vi "Configure Set Vol.vi"(8 "error in (no error)":errorcluster, 9 "Voltage set (0.00 V)":dbl format="%.2g", 10 "Ch Selector":T1, 11 "VISA resource name":refnum<visa-resource-name>) -> (0 "error out":errorcluster, 3 "VISA resource name out":refnum<visa-resource-name>)   [LabVIEW 2020, in "ScientiFic DC Power Supply.lvlib"]
doc: "Configures Set voltage of the power supply. Specify the set voltage limit for Your Application"
uses:
  <instrlib>/ScientiFic DC Power Supply/ScientiFic DC Power Supply.lvlib
  <instrlib>/ScientiFic DC Power Supply/Public/Ch Selector.ctl
panel:
  out "read buffer":string
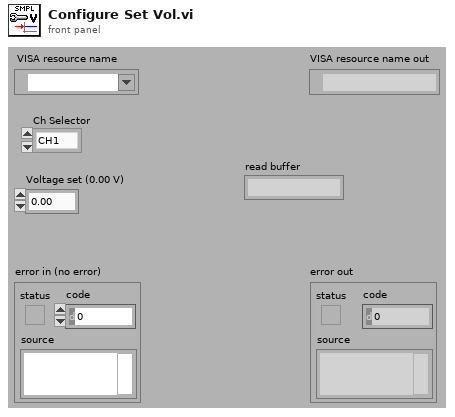
[diagram p1: front panel]
types:
  T1 = typedef "ScientiFic DC Power Supply.lvlib/Ch Selector.ctl" = enum16{"CH1", "CH2", "CH3", "CH4"}
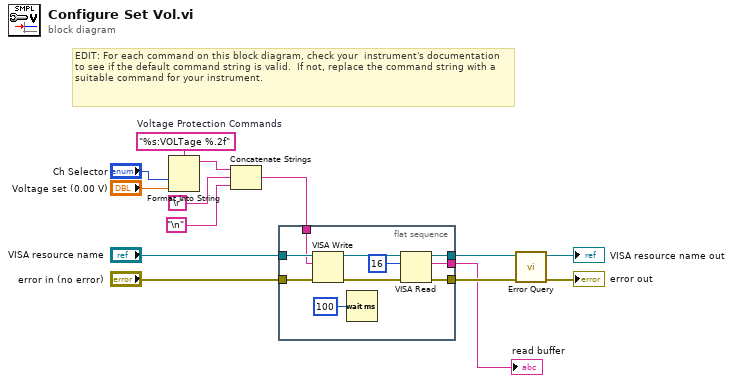
[diagram p0: block diagram]
diagram:
  w10 = "%s:VOLTage %.2f"  # Voltage Protection Commands
  # "EDIT: For each command on this block diagram, check your  instrument's documentation to see if the default command string is valid.  If not, replace the command string with a suitable command for your instrument."
  n1 = Format Into String(format string=w10, "Ch Selector", "Voltage set (0.00 V)") -> (resulting string=w8:string)  [unwired: 2 in, 1 out]
  n2 = Concatenate Strings(w8, "\r", "\n") -> (w5:string)
  n3 = flat-sequence {
    tunnel: "VISA resource name" -> [w23]
    tunnel: "error in (no error)" -> [w22]
    tunnel: w5 -> [w21]
    tunnel: [w20] -> w4
    tunnel: [w18] -> w3
    tunnel: [w16] -> w2
    frame #0 {
      n4 = VISA Write(VISA resource name=w23, write buffer=w21, error in (no error)=w22) -> (VISA resource name out=w24:refnum<visa-resource-name>, error out=w19:errorcluster)  [unwired: 1 out]
      n5 = Wait (ms)(milliseconds to wait=u32 100) -> ()  [unwired: 1 out]
      n6 = VISA Read(VISA resource name=w24, byte count=u32 16, error in (no error)=w19) -> (VISA resource name out=w20:refnum<visa-resource-name>, read buffer=w16:string, error out=w18:errorcluster)  [unwired: 1 out]
    }
  }
  n7 = call <instrlib>:"Error Query.vi"("error in (no error)"=w3, "VISA resource name"=w4) -> ("error out"=→"error out":errorcluster, "VISA resource name out"=→"VISA resource name out":refnum<visa-resource-name>)  [unwired: 8 in]
  "read buffer" <- w2
